vi "Getting Started.vi"() -> ()   [LabVIEW 2014]
uses:
  <vilib>/Motion/plugins/PluginFramework/nismSDIFramework.SetFrameworkMode.single.vi
  <vilib>/Motion/Express/_s/nimc.ex.clearFaults.clearFaults.axis.vi
  <vilib>/Motion/Express/_s/nimc.ex.power.power.axis.vi
  <vilib>/Motion/Express/_s/nimc.ex.straightLineMove.startStraightLineMove.axis.modeRelative.0.vi
  <vilib>/Motion/BlockNode/FB.NIMotion.xnode
  <vilib>/Motion/plugins/Delta SDI Plug-in/Template SoftMotion Drive Interface Plug-in Class.lvclass
panel:
  in  "Motion Resource":refnum<k21>="Axis 1"
  in  "velocity":dbl=1000000.0
  in  "position":dbl=1024000.0
  out "error out":errorcluster
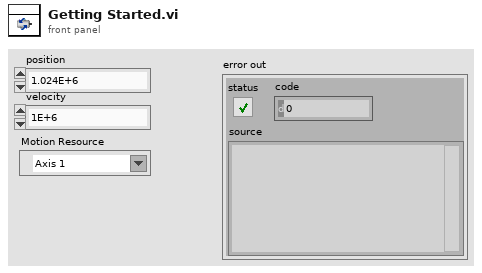
[diagram p1: front panel]
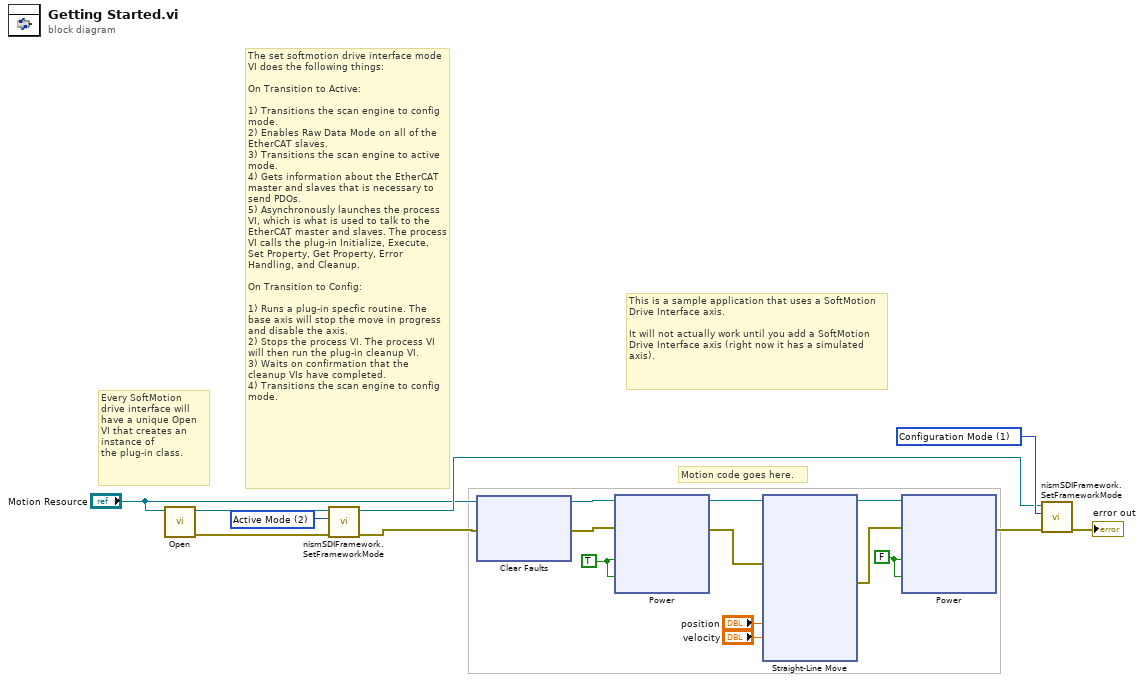
[diagram p0: block diagram]
diagram:
  w3 = FALSE ("enable axis")
  w10 = TRUE ("enable axis")
  w18 = 1 items=["Configuration Mode"=1, "Active Mode"=2] ("mode (Active Mode)")
  w19 = 2 items=["Configuration Mode"=1, "Active Mode"=2] ("mode (Active Mode)")
  # "Motion code goes here."
  # "The set softmotion drive interface mode VI does the following things:\n\nOn Transition to Active:\n\n1) Transitions the scan engine to config mode.\n2) Enables Raw Data Mode on all of the EtherCAT slaves.\n3) Transitions the scan engine to active mode.\n4) Gets information about the EtherCAT master and slaves that is necessary to send PDOs.\n5) Asynchronously launches the process VI, which is what is used to talk to the EtherCAT master and slaves. The process VI calls the plug-in Initialize, Execute, Set Property, Get Property, Error Handling, and Cleanup.\n\nOn Transition to Config:\n\n1) Runs a plug-in specfic routine. The base axis will stop the move in progress and disable the axis.\n2) Stops the process VI. The process VI will then run the plug-in cleanup VI.\n3) Waits on confirmation that the cleanup VIs have completed.\n4) Transitions the scan engine to config mode."
  # "Every SoftMotion drive interface will have a unique Open VI that creates an instance of\nthe plug-in class."
  # "This is a sample application that uses a SoftMotion Drive Interface axis.\n\nIt will not actually work until you add a SoftMotion Drive Interface axis (right now it has a simulated axis)."
  n1 = call <vilib>:"Open.vi"("Axis"="Motion Resource") -> ("error out"=w12:errorcluster, "Base Axis Out"=w13:refnum<class "nismPluginAxisBaseClass.lvclass">)  [unwired: 9 in]
  n2 = call-poly <vilib>:"nismSDIFramework.SetFrameworkMode.vi"("error in (no error)"=w12, "mode (Active Mode)"=w19, "Base Axis In"=w13) -> ("error out"=w15:errorcluster, "Base Axis Out"=w16:refnum<class "nismPluginAxisBaseClass.lvclass">)  [unwired: 7 in]
  n3 = xnode ("Clear Faults")("resource"="Motion Resource", "error in"=w15) -> ("resource out"=w2:refnum<k21>, "error out"=w1:errorcluster)
  n4 = xnode ("Power")("enable axis"=w10, "enable drive"=w10, "resource"=w2, "error in"=w1) -> ("resource out"=w8:refnum<k21>, "error out"=w9:errorcluster)
  n5 = xnode ("Straight-Line Move")("position"="position", "velocity"="velocity", "resource"=w8, "error in"=w9) -> ("resource out"=w5:refnum<k21>, "error out"=w4:errorcluster)  [unwired: 6 in, 1 out]
  n6 = xnode ("Power")("enable axis"=w3, "enable drive"=w3, "resource"=w5, "error in"=w4) -> ("error out"=w17:errorcluster)  [unwired: 1 out]
  n7 = call-poly <vilib>:"nismSDIFramework.SetFrameworkMode.vi"("error in (no error)"=w17, "mode (Active Mode)"=w18, "Base Axis In"=w16) -> ("error out"=→"error out":errorcluster)  [unwired: 7 in, 1 out]
